vi "Get Maximum Power.vi"(0 "COM Port in":refnum<visa-resource-name>, 1 "error in":errorcluster) -> (2 "COM Port out":refnum<visa-resource-name>, 3 "maximum power":i32, 4 "OK":bool, 5 "error out":errorcluster)   [LabVIEW 2013]
doc: "This command gives back the truly maximum available power of the laser/led system.\n\nThis parameter may differ from the “Spec Power” parameter. For example if a laser is equipped with a direct fiber output option you will not reach the specified power after the fiber because of damping issues. Since we are interested in the power of the whole laser system the maximum power will be slightly below the specified diode power."
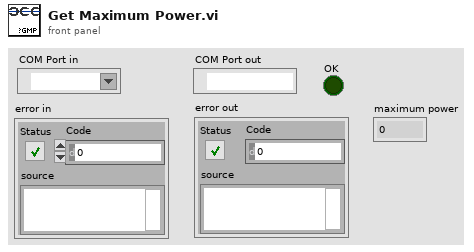
[diagram p1: front panel]
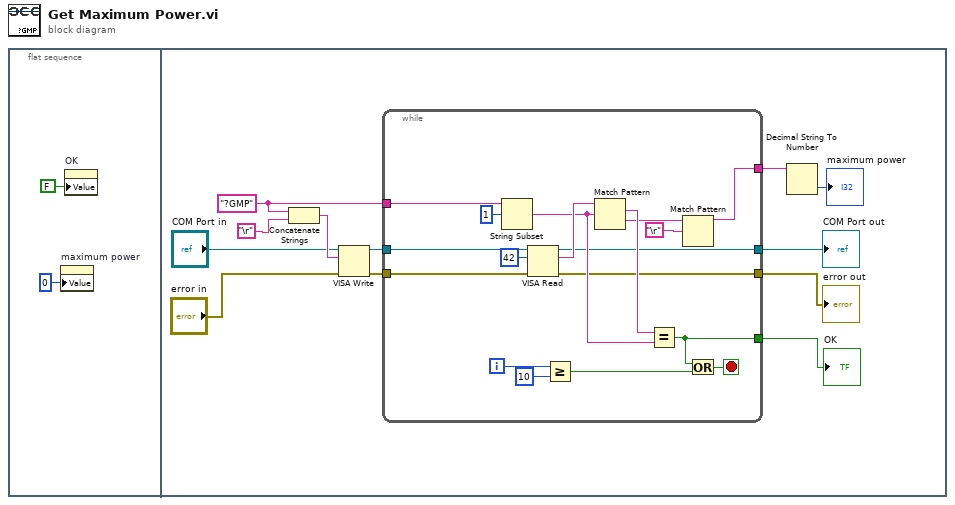
[diagram p0: block diagram]
diagram:
  n1 = flat-sequence {
    frame #0 {
      n2 = property on="maximum power" class="DigWert (strikt)"("Value"=0 ("maximum power")) -> ()  [unwired: 2 in, 2 out]
      n3 = property on="OK" class="Bool. (strikt)"("Value"=FALSE ("OK")) -> ()  [unwired: 2 in, 2 out]
    }
    frame #1 {
      w8 = "?GMP" ("Schreibpuffer")
      n4 = Concatenate Strings(w8, "\r") -> (w10:string)
      n5 = VISA Write(VISA resource name="COM Port in", write buffer=w10, error in (no error)="error in") -> (VISA resource name out=w4:refnum<visa-resource-name>, error out=w5:errorcluster)  [unwired: 1 out]
      n6 = while {
        tunnel: [w27] -> w14
        tunnel: [w26] -> w13
        tunnel: [w22] -> w12
        tunnel: w8 -> [w19]
        tunnel: w5 -> [w18]
        tunnel: w4 -> [w16]
        tunnel: [w17] -> w3
        i -> [w25]
        stop <- w20 stop-if-true
        n7 = String Subset(string=w19, offset (0)=1 ("Offset (0)")) -> (substring=w28:string)  [unwired: 1 in]
        n8 = VISA Read(VISA resource name=w16, byte count=u32 42 ("Byte-Anzahl"), error in (no error)=w18) -> (VISA resource name out=w27:refnum<visa-resource-name>, read buffer=w31:string, error out=w26:errorcluster)  [unwired: 1 out]
        n9 = Greater Or Equal?(x=w25, y=10) -> (x >= y?=w23:bool)
        n10 = Match Pattern(string=w31, regular expression=w28) -> (match substring=w30:string, after substring=w21:string)  [unwired: 1 in, 2 out]
        n11 = Equal?(x=w30, y=w28) -> (x = y?=w17:bool)
        n12 = Match Pattern(string=w21, regular expression="\r") -> (before substring=w22:string)  [unwired: 1 in, 3 out]
        n13 = Or(x=w17, y=w23) -> (x .or. y?=w20:bool)
      }
      "COM Port out" <- w14
      "error out" <- w13
      "OK" <- w3
      n14 = Decimal String To Number(string=w12) -> (number=→"maximum power":i32)  [unwired: 2 in, 1 out]
    }
  }
